vi "CR-导丝颗粒物检测2.vi"(8 "error in (no error)":errorcluster caption="错误输入（无错误）", 11 "名称或相对路径":string="Template Program") -> (0 "error in (no error) 2":errorcluster caption="错误输入（无错误）")   [LabVIEW 2017]
uses:
  Global System.vi
  <vilib>/Utility/xml.llb/Write to XML File(string).vi
  Picture/SaveButtom.ctl
  <vilib>/userdefined/High Color/IMAQdx.ctl
panel:
  in  "相机选择":T1="cam0" caption="Session Out CCD3"
  in  "获取图像":bool
  in  "ROI获取":bool
  in  "创建模板":bool
  in  "保存图像":bool
  out "添加的路径":path
  in  "刷新":bool
  in  "测试按钮":bool
  in  "保存按钮":bool
  in  "Main":enum32{"主参数", "模板匹配参数 ", "测试效果"}(tab)
  in  "颗粒物检测2基础参数":T2={"IsNorImage"=TRUE, "Exposure Values"=100289, "ImagePath"=path "C:/Users/hedongpo/Desktop/514-hdp/Alignment Assemble System/Test Picture/B/3.bmp"} caption="参数界面" {"Exposure Values" scale=0.0..200000.0}
  in  "颗粒物检测2参数":T4={"Rectangle"={"Left"=0, "Top"=0, "Right"=0, "Bottom"=0, "Rotation"=0.0}, "Threshold Limits (Threshold 1)"={"Lower value"=6.0, "Upper value"=245.0}, "Keep/Remove Particles "=FALSE, "Connectivity 4/8 (8) "=TRUE, "Selection Values (Particle Filter 1)"=[{"Measurement Parameter"=35, "Range Lower Value"=80.0, "Range Upper Value"=16332.0, "Range"=FALSE, "Measurement Type"=FALSE}], "Corner Options (Feature Detection 1)"={"Detector type"=enum."Harris Corner", "Kernel size"=7, "Min Corner Point Strength"=32.0}, "Pyramid level (Feature Detection 1)"=3, "Method "=2, "Look For"=0, "Method 2"=2, "ROI Descriptor (Clamp (Rake) 1)"={"Global Rectangle"=[162, 394, 420, 1807], "Contours"=[{"ID"=enum."External", "Type"=12, "Coordinates"=[162, 394, 420, 1807, 0]}]}} {"Method" items=["clustering", "entropy", "metric", "moments", "inter-class variance"]; "Look For" items=["Bright Objects", "Dark Objects"]; "Method 2" items=["clustering", "entropy", "metric", "moments", "inter-class variance"]; "ROI Descriptor (Clamp (Rake) 1)"."Contours"."Type" items=["No Selection", "Point", "Line", "Rectangle", "Oval", "Polygon", "Freehand Region", "Annulus", "Unused2", "Unused3", "Broken Line", "Freehand Line", "Rotated Rectangle"]; "Selection Values (Particle Filter 1)"."Measurement Parameter" items=["Center of Mass X", "Center of Mass Y", "First Pixel X", "First Pixel Y", "Bounding Rect Left", "Bounding Rect Top", "Bounding Rect Right", "Bounding Rect Bottom", "Max Feret Diameter Start X", "Max Feret Diameter Start Y", "Max Feret Diameter End X", "Max Feret Diameter End Y", "Max Horiz. Segment Length Left", "Max Horiz. Segment Length Right", "Max Horiz. Segment Length Row", "-", "Bounding Rect Width", "Bounding Rect Height", "Bounding Rect Diagonal", "Perimeter", "Convex Hull Perimeter", "Holes' Perimeter", "Max Feret Diameter", "Equivalent Ellipse Major Axis", "Equivalent Ellipse Minor Axis", "Equivalent Ellipse Minor Axis (Feret)", "Equivalent Rect Long Side", "Equivalent Rect Short Side", "Equivalent Rect Diagonal", "Equivalent Rect Short Side (Feret)", "Average Horiz. Segment Length", "Average Vert. Segment Length", "Hydraulic Radius", "Waddel Disk Diameter", "-", "Area", "Holes' Area", "Particle & Holes' Area", "Convex Hull Area", "Image Area", "-", "Number of Holes", "Number of Horiz. Segments", "Number of Vert. Segments", "-", "Orientation", "Max Feret Diameter Orientation", "-", "% Area/Image Area", "% Area/(Particle & Holes' Area)", "Ratio of Equivalent Ellipse Axes", "Ratio of Equivalent Rect Sides", "-", "Elongation Factor", "Compactness Factor", "Heywood Circularity Factor", "Type Factor", "-", "Sum X", "Sum Y", "Sum XX", "Sum XY", "Sum YY", "Sum XXX", "Sum XXY", "Sum XYY", "Sum YYY", "-", "Moment of Inertia XX", "Moment of Inertia XY", "Moment of Inertia YY", "Moment of Inertia XXX", "Moment of Inertia XXY", "Moment of Inertia XYY", "Moment of Inertia YYY", "Norm. Moment of Inertia XX", "Norm. Moment of Inertia XY", "Norm. Moment of Inertia YY", "Norm. Moment of Inertia XXX", "Norm. Moment of Inertia XXY", "Norm. Moment of Inertia XYY", "Norm. Moment of Inertia YYY", "Hu Moment 1", "Hu Moment 2", "Hu Moment 3", "Hu Moment 4", "Hu Moment 5", "Hu Moment 6", "Hu Moment 7"]; "Rectangle"."Rotation" min=-90.0 max=90.0 step=1.0 format="%.2f"; "Rectangle"."Left" scale=0.0..1024.0; "Rectangle"."Right" scale=0.0..1024.0}
  in  "Feature Points Strength":string[][](table)
  out "原始图像":T5(plugin-control)
  out "颗粒物有无显示":bool
  out "Number of Features Found":i32
  in  "颗粒物个数阈值":i32
  out "路径输出":path
  in  "Vision Paramter Save Buttom":T6
  out "system time":string
  in  "取消按钮":bool
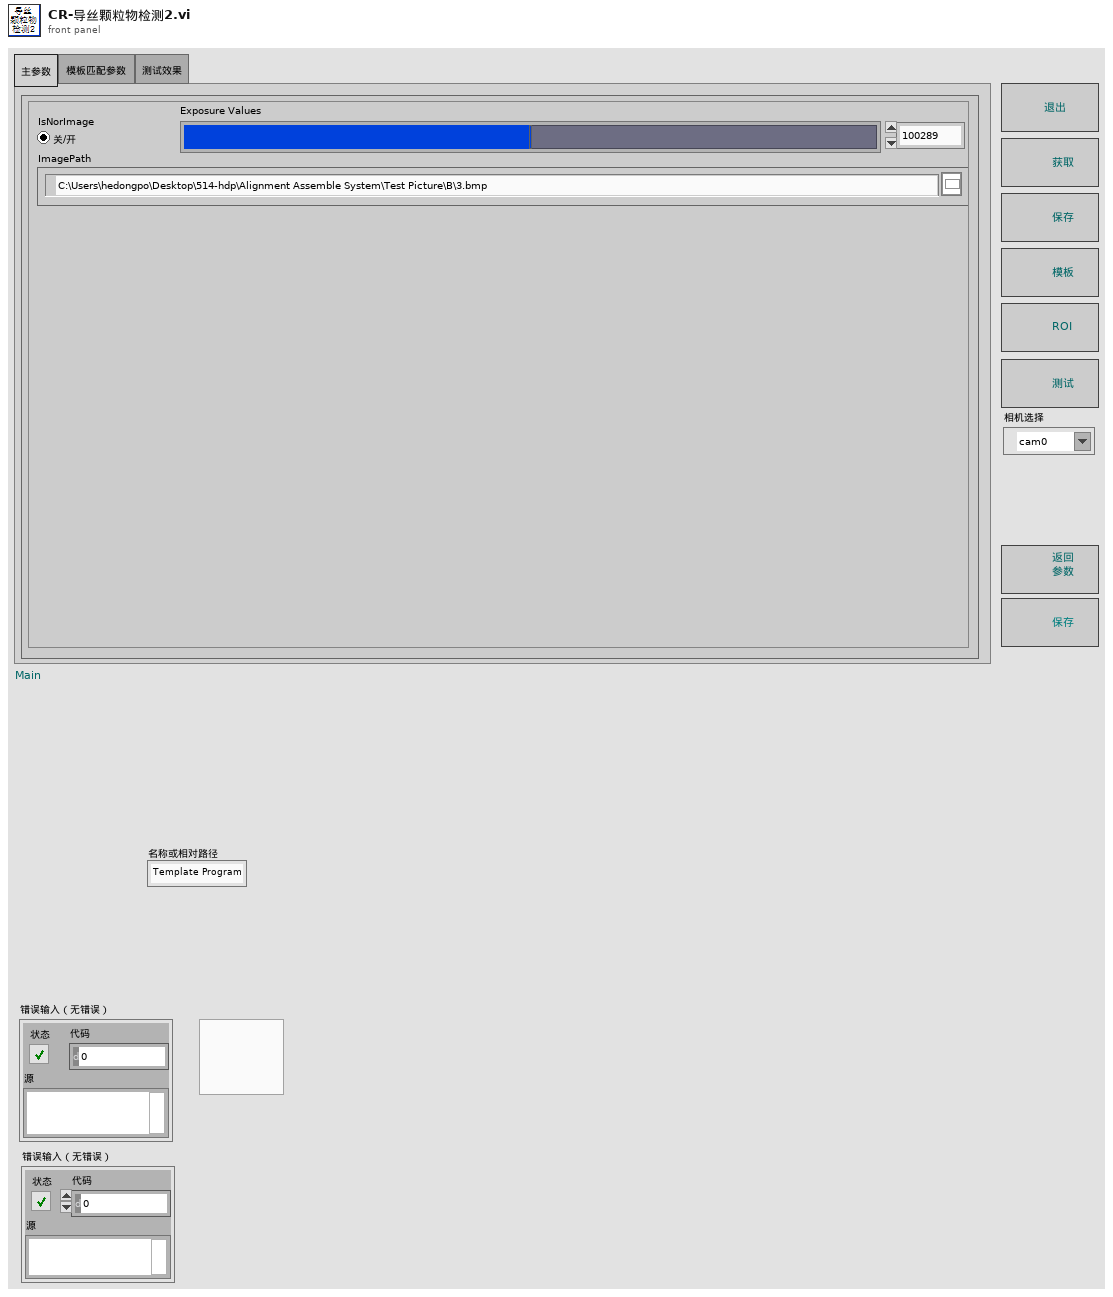
[diagram p1: front panel]
types:
  T1 = typedef "IMAQdx.ctl" = refnum<k21>
  T2 = cluster{"IsNorImage":bool, "Exposure Values":u32, "ImagePath":path}
  T3 = typedef "IMAQ Rectangle" = cluster{"Left":i32, "Top":i32, "Right":i32, "Bottom":i32, "Rotation":dbl}
  T4 = cluster{"Rectangle":T3, "Threshold Limits (Threshold 1)":cluster{"Lower value":sgl, "Upper value":sgl}, "Keep/Remove Particles ":bool, "Connectivity 4/8 (8) ":bool, "Selection Values (Particle Filter 1)":cluster{"Measurement Parameter":i32, "Range Lower Value":dbl, "Range Upper Value":dbl, "Range":bool, "Measurement Type":bool}[], "Corner Options (Feature Detection 1)":cluster{"Detector type":enum32{"Harris Corner", "Shi-Tomasi Corner"}, "Kernel size":i32, "Min Corner Point Strength":dbl}, "Pyramid level (Feature Detection 1)":u32, "Method ":i32, "Look For":u32, "Method 2":i32, "ROI Descriptor (Clamp (Rake) 1)":cluster{"Global Rectangle":i32[], "Contours":cluster{"ID":enum32{"External", "Internal"}, "Type":u32, "Coordinates":i32[]}[]}}
  T5 = typedef "IMAQ Image.ctl" = refnum<image>
  T6 = typedef "SaveButtom.ctl" = bool
  T7 = cluster{"index":i32, "this vi":refnum<vi>, "error out":errorcluster}
  T8 = cluster{"master data":string, "priority":u16, "secondary data":string[]}
  T9 = cluster{"case name":string[], "queue array":refnum<queue>[]}
  T10 = cluster{"Global Rectangle":i32[], "Contours":cluster{"Contour Type":u32, "ROI Type":u32, "Points":i32[]}[]}
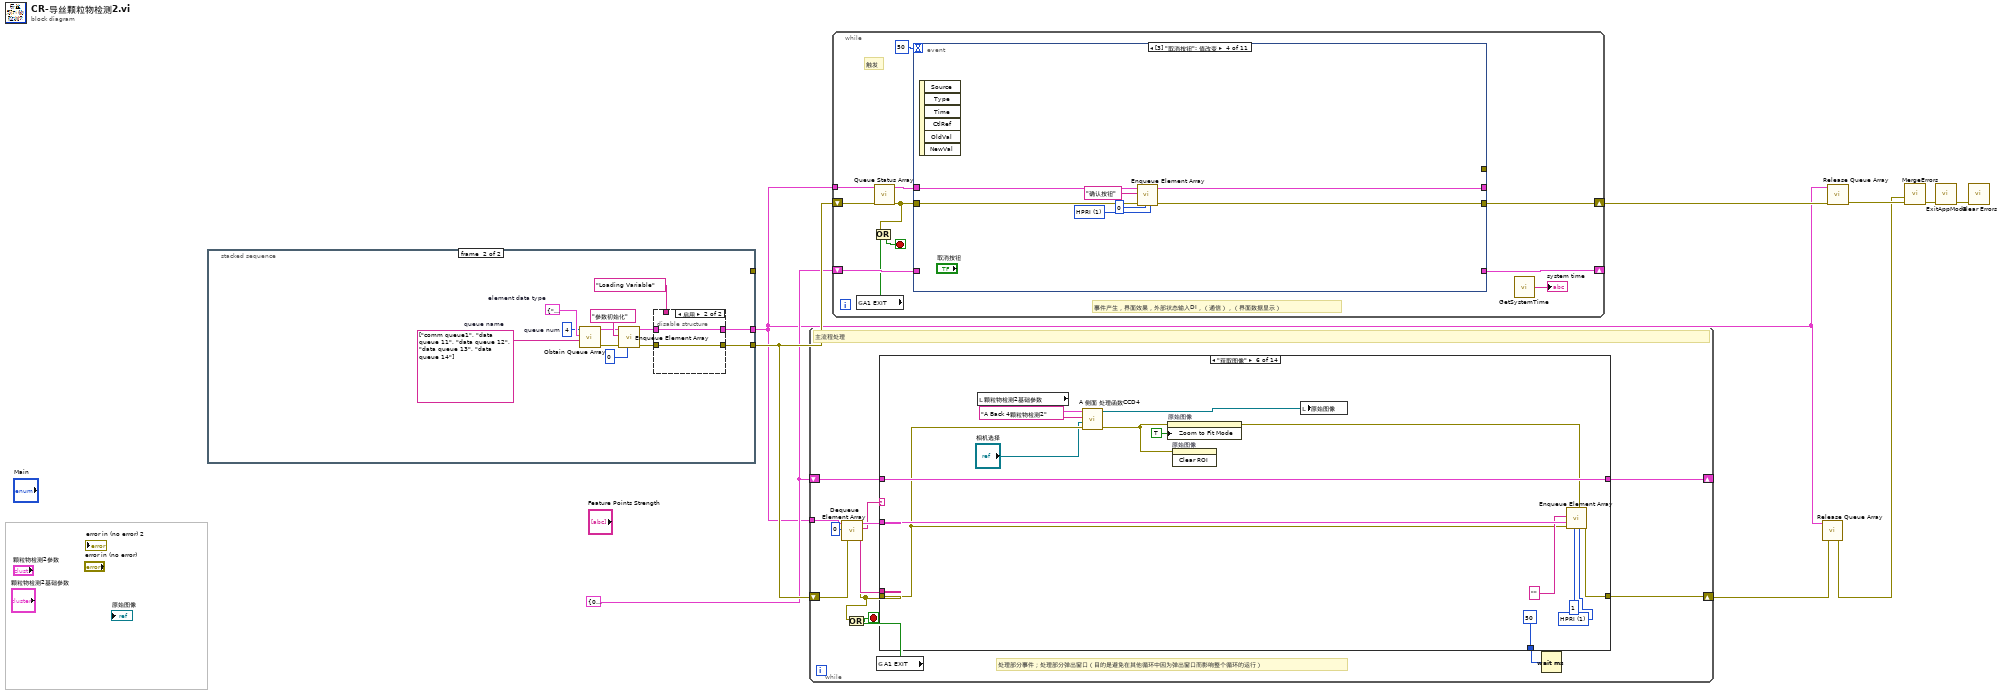
[diagram p0: block diagram]
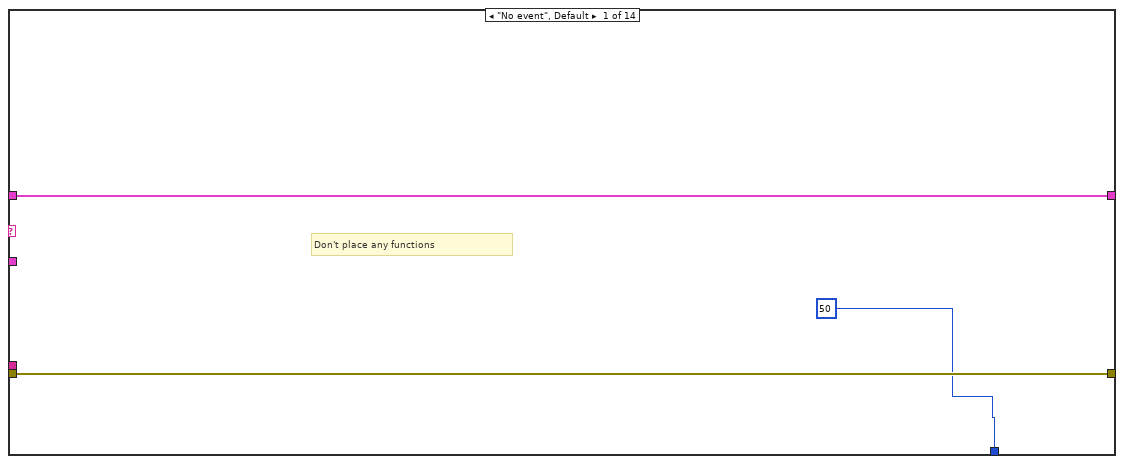
[diagram p2: hidden frame]
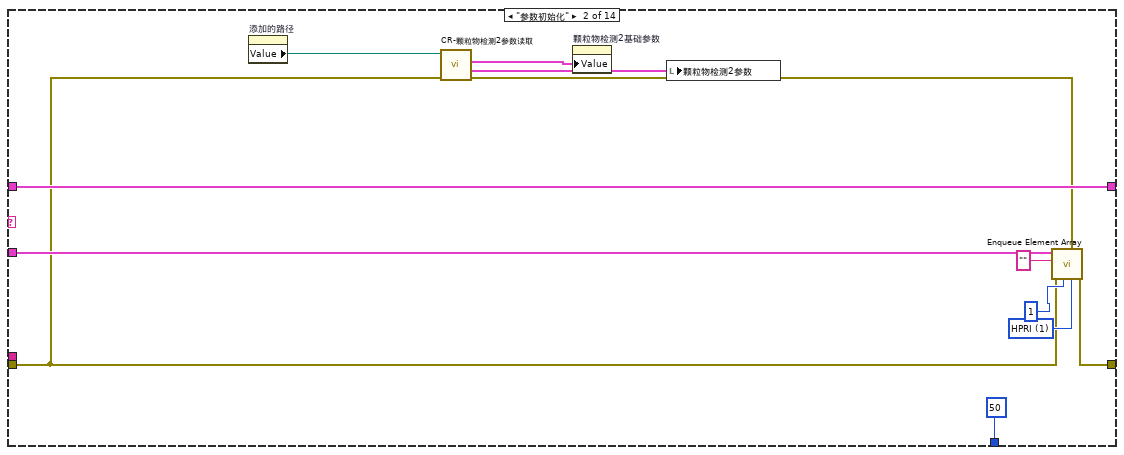
[diagram p3: hidden frame]
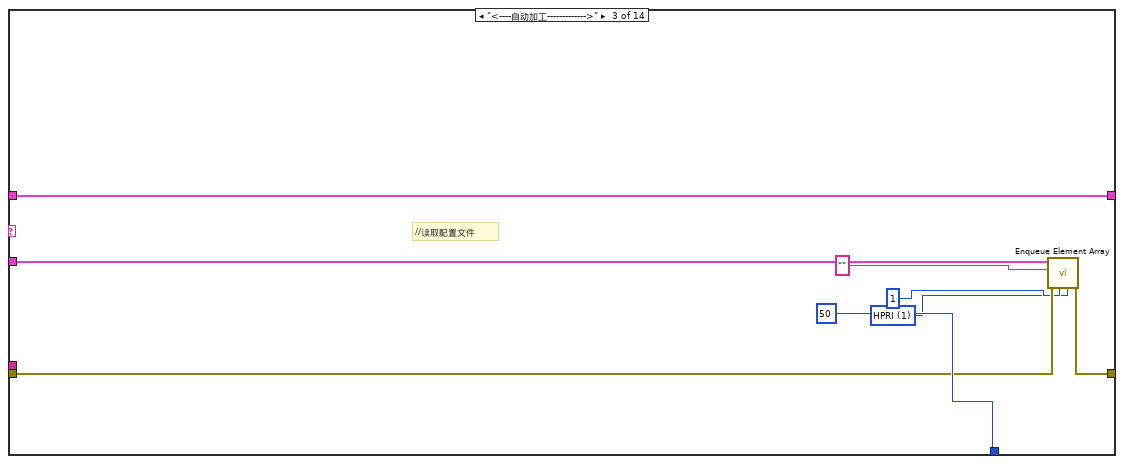
[diagram p4: hidden frame]
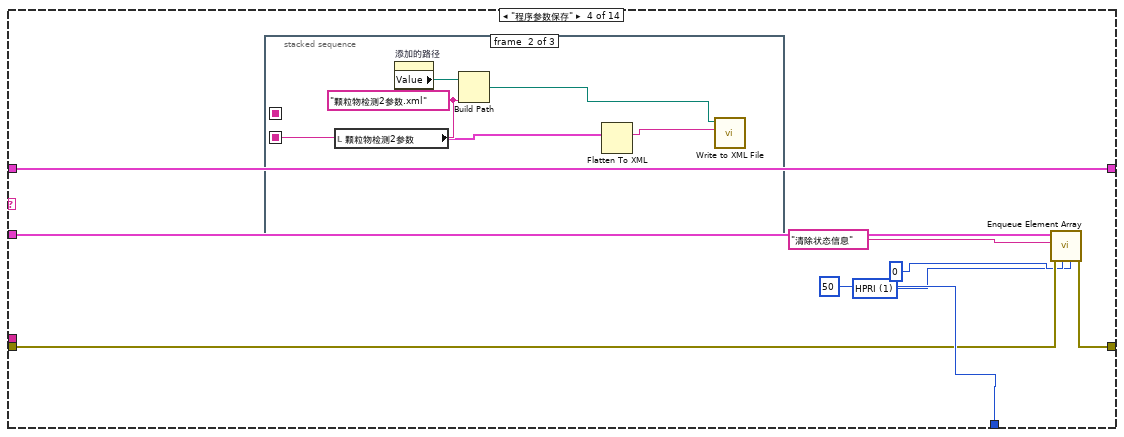
[diagram p5: hidden frame]
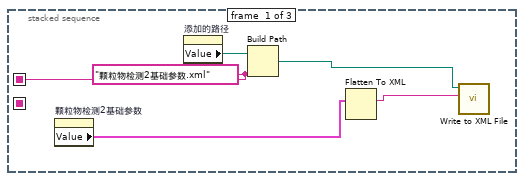
[diagram p6: hidden frame]
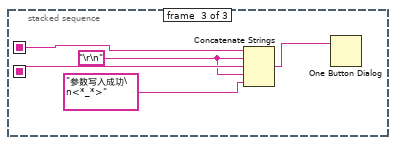
[diagram p7: hidden frame]
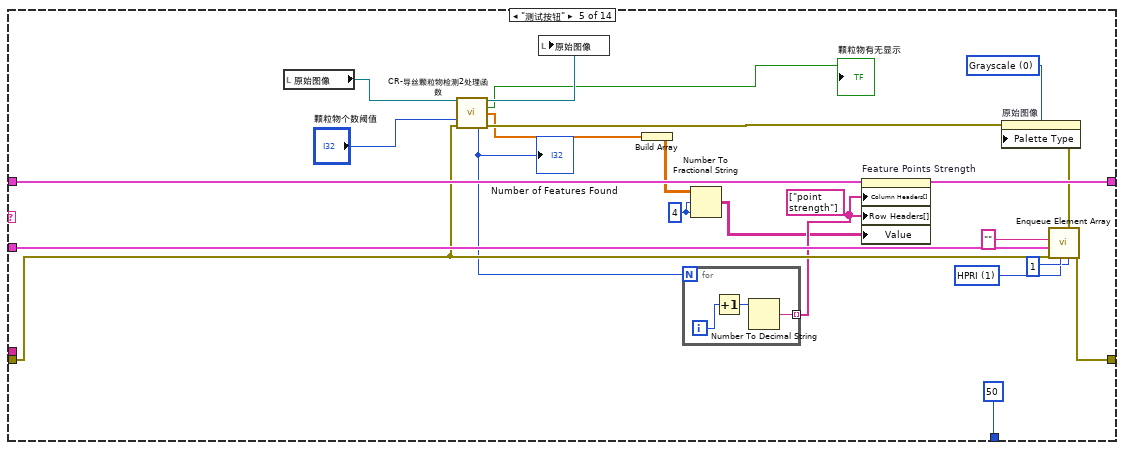
[diagram p8: hidden frame]
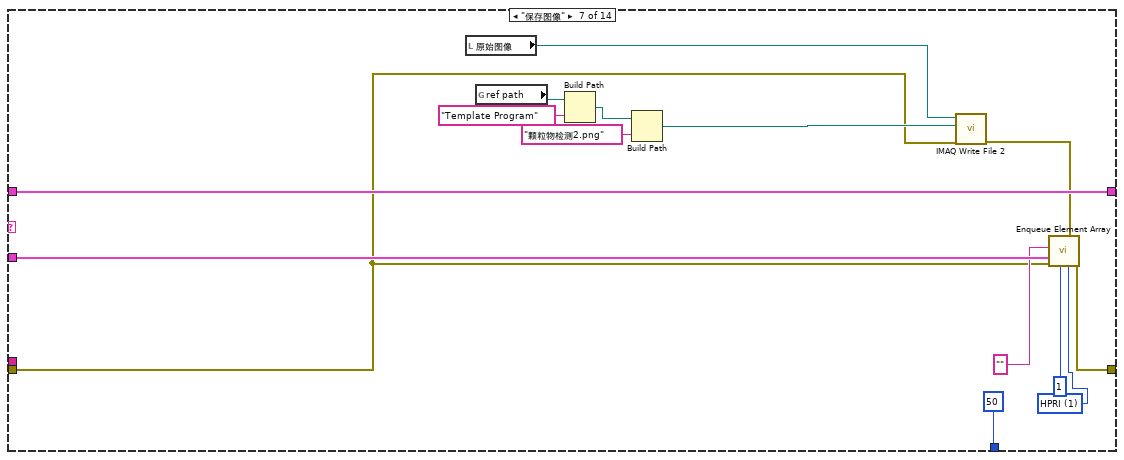
[diagram p9: hidden frame]
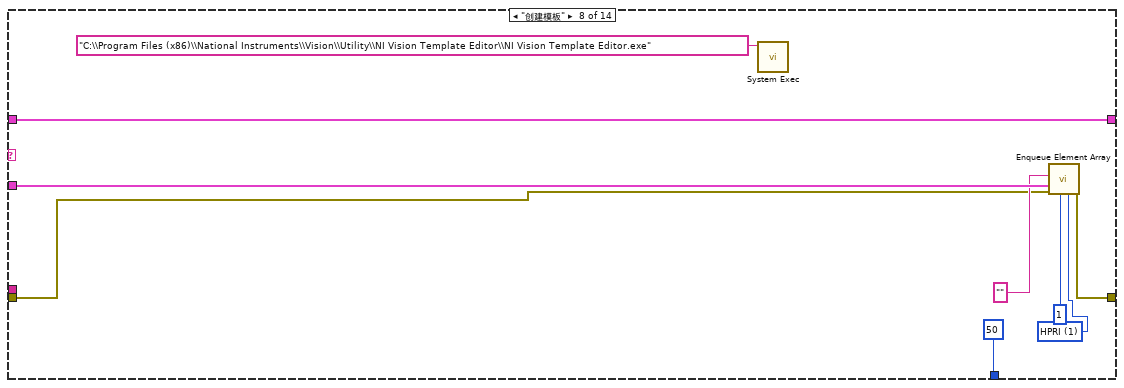
[diagram p10: hidden frame]
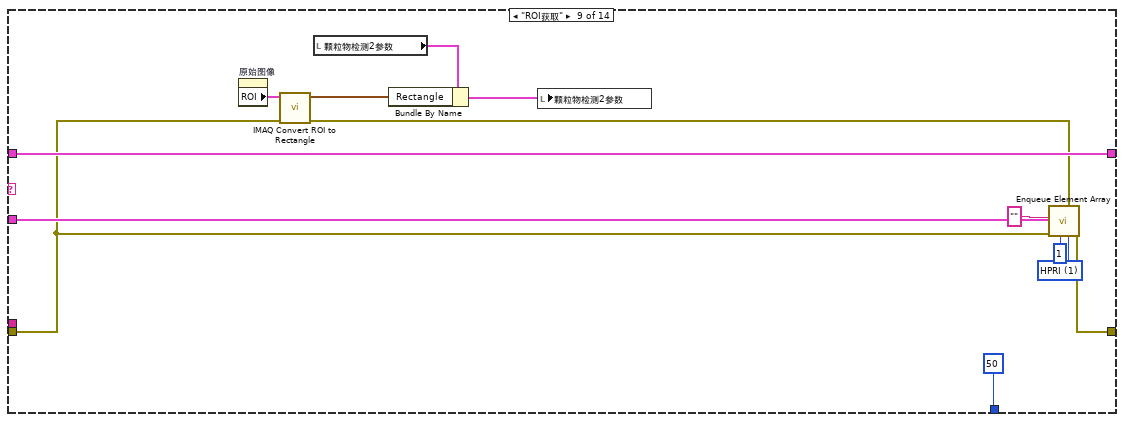
[diagram p11: hidden frame]
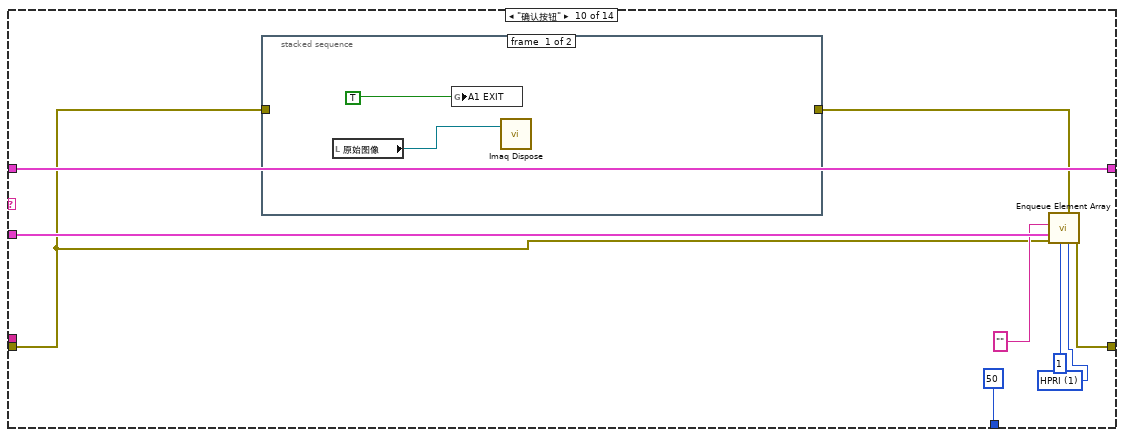
[diagram p12: hidden frame]
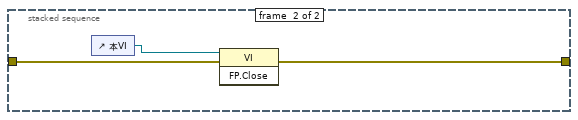
[diagram p13: hidden frame]
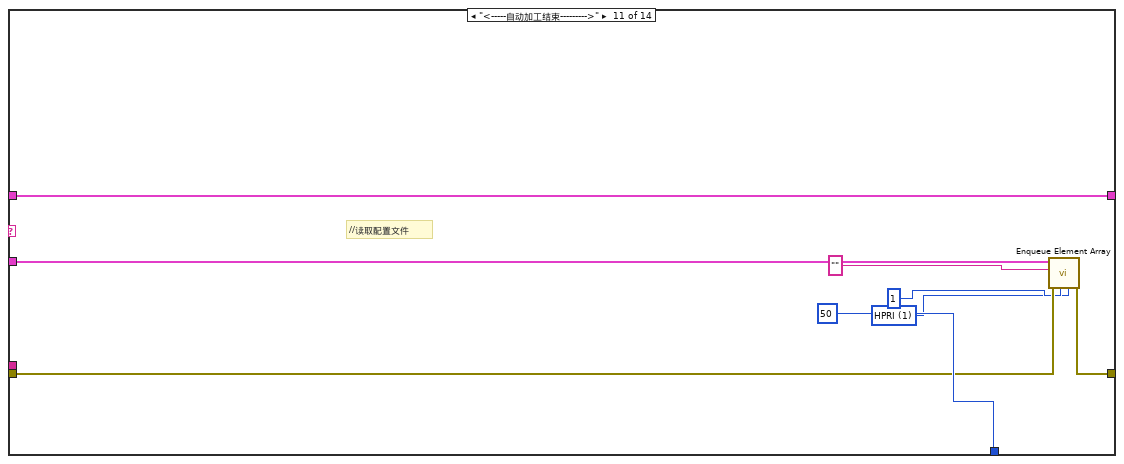
[diagram p14: hidden frame]
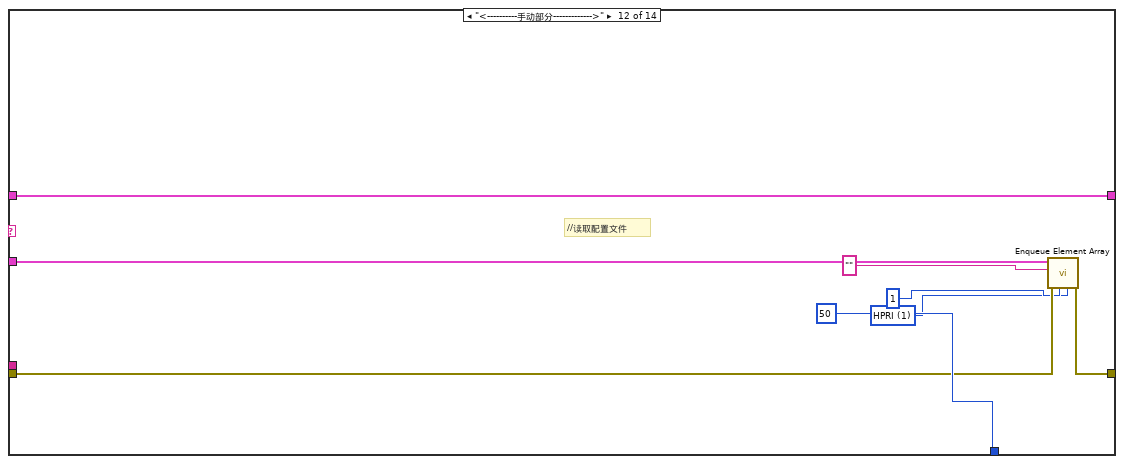
[diagram p15: hidden frame]
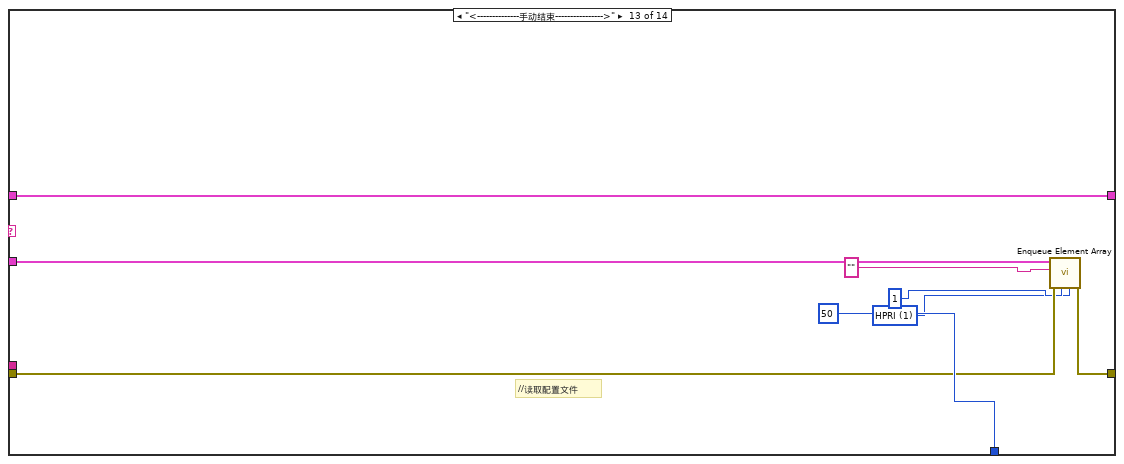
[diagram p16: hidden frame]
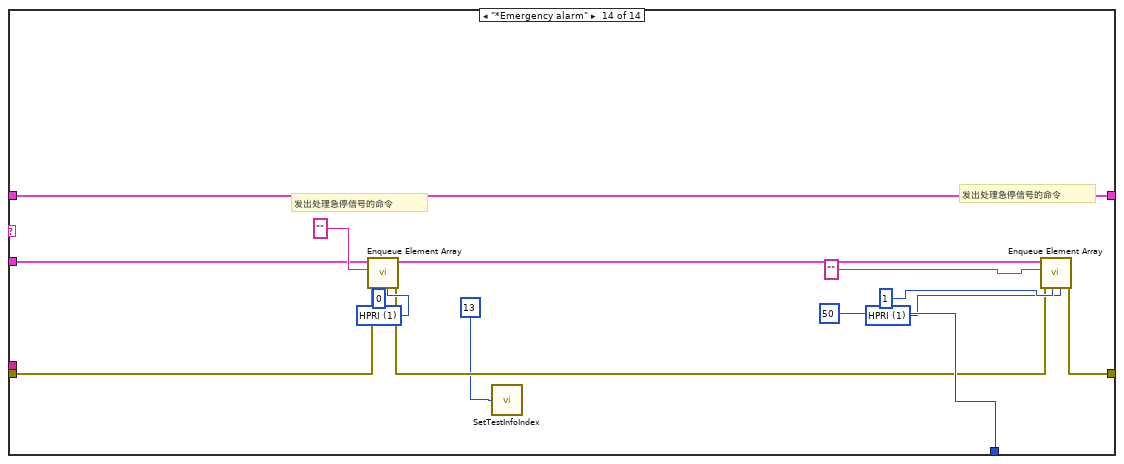
[diagram p17: hidden frame]
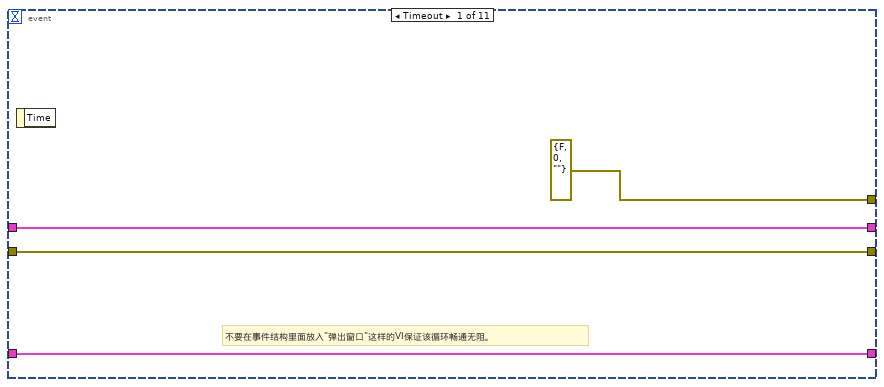
[diagram p18: hidden frame]
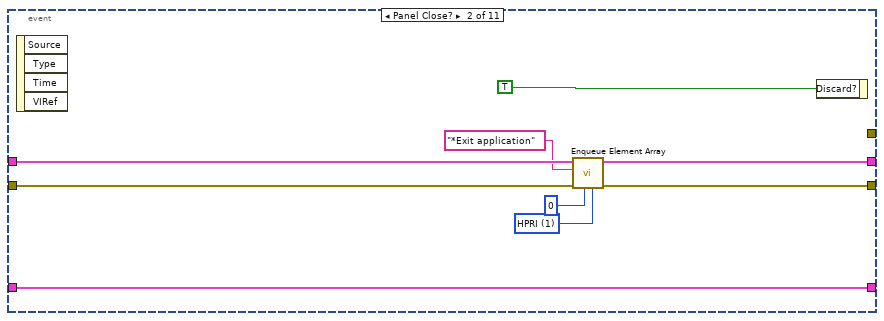
[diagram p19: hidden frame]
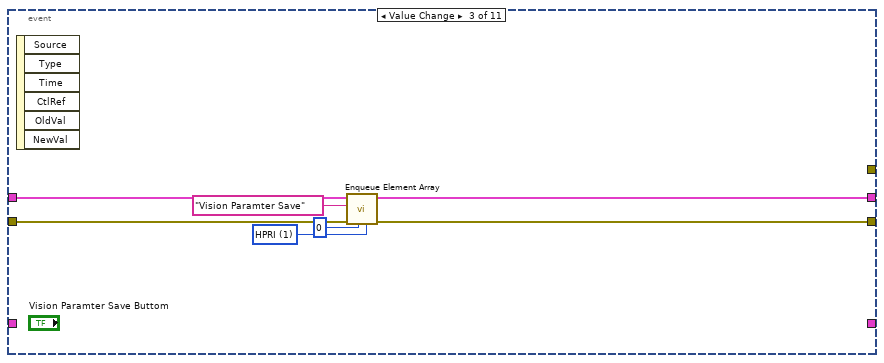
[diagram p20: hidden frame]
diagram:
  w4 = T7 {"index"=0, "this vi"=refnum, "error out"={"status"=FALSE, "code"=0, "source"=""}} ("parameter buffer")
  n1 = stacked-sequence {
    tunnel: [w15 _] -> _
    tunnel: [_ w19] -> w5
    tunnel: [_ w18] -> w1
    frame #0 {
      n2 = global read "Global System.vi" "ref path"() -> (w13:path)
      n3 = Build Path(base path=w13, name or relative path="Template Program" ("名称或相对路径")) -> (appended path=w11:path)
      n4 = property on="Main" class="TabCtl (严格)"("Value"=enum32{"主参数", "模板匹配参数 ", "测试效果"}."主参数" ("Main")) -> ()  [unwired: 2 in, 2 out]
      n5 = Build Path(base path=w11, name or relative path="名称或相对路径") -> (appended path=w17:path)
      "添加的路径" <- w17
      n6 = List Folder(path=w17) -> (path out=→"路径输出":path, error out=w15:errorcluster)  [unwired: 3 in, 2 out]
    }
    frame #1 {
      w27 = string[] ["comm queue1", "data queue 11", "data queue 12", "data queue 13", "data queue 14"]  # queue name
      w28 = 4  # queue num
      w29 = T8 {"master data"="", "priority"=0, "secondary data"=[]}  # element data type
      n7 = call "Obtain Queue Array.vi"("queue name"=w27, "element data type"=w29, "queue num"=w28) -> ("error out"=w23:errorcluster, "queue out"=w24:T9)  [unwired: 2 in, 1 out]
      n8 = call "Enqueue Element Array.vi"("queue index"=0, "error in"=w23, "master data"="参数初始化", "queue in"=w24) -> ("error out"=w22:errorcluster, "queue out"=w21:T9)  [unwired: 6 in]
      n9 = disable-structure shown="启用" {
        disable-tunnel: w22 -> [w35 w36]
        disable-tunnel: w21 -> [w34 w37]
        disable-tunnel: "Loading Variable" ("master data") -> [w33 _]
        disable-tunnel: [w31 w36] -> w19
        disable-tunnel: [w30 w37] -> w18
        frame Disabled {
          n10 = call "Enqueue Element Array.vi"("queue index"=12, "error in"=w35, "master data"=w33, "queue in"=w34) -> ("error out"=w31:errorcluster, "queue out"=w30:T9)  [unwired: 6 in]
        }
        frame Enabled {
        }
      }
    }
  }
  n11 = while {
    shift-right: [w50] -> w3
    shift-left: w5 -> [w41]
    shift-right: [w47] -> _
    shift-left: w4 -> [w48]
    tunnel: w1 -> [w43]
    stop <- w38 stop-if-true
    # "处理部分事件；处理部分弹出窗口（目的是避免在其他循环中因为弹出窗口而影响整个循环的运行）"
    # "主流程处理"
    n12 = call "Dequeue Element Array.vi"("queue in"=w43, "queue index"=0, "error in"=w41) -> ("queue out"=w46:T9, "master data"=w45:string, "secondary data"=w44:string[], "error out"=w40:errorcluster)  [unwired: 2 in, 1 out]
    n13 = global read "Global System.vi" "A1 EXIT"() -> (w39:bool)
    n14 = Or(x=w40, y=w39) -> (x .or. y?=w38:bool)
    n15 = case shown="\"获取图像\"" w45 {
      tunnel: w46 -> [_ w64 w72 w74 w116 w134 w149 w158 w171 w180 w193 w201 w209 w215]
      tunnel: w40 -> [w52 w57 w68 w78 w110 w125 w136 w152 w164 w174 w189 w197 w205 w212]
      tunnel: [w52 w63 w71 w80 w115 w133 w148 w157 w170 w179 w192 w200 w208 w223] -> w50
      tunnel: [50 50 50 50 50 50 50 50 50 50 50 50 50 50] -> w49
      tunnel: w48 -> [w53 w59 w69 w75 w111 w129 w144 w153 w166 w175 w190 w198 w206 w221]
      tunnel: [w53 w59 w69 w75 w111 w129 w144 w153 w166 w175 w190 w198 w206 w221] -> w47
      tunnel: w44 -> [_ _ _ _ _ _ _ _ _ _ _ _ _ _]
      frame "No event", Default {
        # "Don't place any functions"
      }
      frame "参数初始化" {
        w60 = u16 1 items=["HPRI"=1, "LPRI"=0] ("priority")
        n16 = property on="添加的路径" class="Path"() -> ("Value"=w58:path)  [unwired: 2 in, 2 out]
        n17 = call "CR-颗粒物检测2参数读取.vi"("error in (no error)"=w57, "基路径"=w58) -> ("error out"=w54:errorcluster, "颗粒物检测2参数"=w56:T4, "颗粒物检测2基础参数"=w55:T2)  [unwired: 6 in]
        n18 = property on="颗粒物检测2基础参数" class="Clust (严格)"("Value"=w55) -> ()  [unwired: 2 in, 2 out]
        n19 = local write "颗粒物检测2参数"(w56) -> ()
        n20 = call "Enqueue Element Array.vi"("priority"=w60, "device error in"=w54, "queue index"=1, "error in"=w57, "master data"="" ("Element 1"), "queue in"=w64) -> ("error out"=w63:errorcluster)  [unwired: 4 in, 1 out]
      }
      frame "<----自动加工------------->" {
        w66 = u16 1 items=["HPRI"=1, "LPRI"=0] ("priority")
        # "//读取配置文件"
        n21 = call "Enqueue Element Array.vi"("priority"=w66, "queue index"=1, "error in"=w68, "master data"="" ("Element 1"), "queue in"=w72) -> ("error out"=w71:errorcluster)  [unwired: 5 in, 1 out]
      }
      frame "程序参数保存" {
        w76 = u16 1 items=["HPRI"=1, "LPRI"=0] ("priority")
        n22 = stacked-sequence {
          seq-local: [w82 _ _] -> [_ _ w95]
          seq-local: [_ w88 _] -> [_ _ w93]
          frame #0 {
            w82 = "颗粒物检测2基础参数.xml" ("名称或相对路径")
            n23 = property on="颗粒物检测2基础参数" class="Clust (严格)"() -> ("Value"=w85:T2)  [unwired: 2 in, 2 out]
            n24 = property on="添加的路径" class="Path"() -> ("Value"=w86:path)  [unwired: 2 in, 2 out]
            n25 = Build Path(base path=w86, name or relative path=w82) -> (appended path=w83:path)
            n26 = Flatten To XML(anything=w85) -> (xml string=w84:string)
            n27 = call-poly <vilib>:"Write to XML File.vi"("XML Input"=w84, "XML File Path"=w83) -> ()  [unwired: 7 in, 3 out]
          }
          frame #1 {
            w88 = "颗粒物检测2参数.xml" ("名称或相对路径")
            n28 = local read "颗粒物检测2参数"() -> (w87:T4)
            n29 = property on="添加的路径" class="Path"() -> ("Value"=w91:path)  [unwired: 2 in, 2 out]
            n30 = Build Path(base path=w91, name or relative path=w88) -> (appended path=w89:path)
            n31 = Flatten To XML(anything=w87) -> (xml string=w90:string)
            n32 = call-poly <vilib>:"Write to XML File.vi"("XML Input"=w90, "XML File Path"=w89) -> ()  [unwired: 7 in, 3 out]
          }
          frame #2 {
            w92 = "\r\n"
            n33 = Concatenate Strings(w95, w92, w93, w92, "参数写入成功\n<*_*>" ("消息")) -> (w94:string)
            n34 = One Button Dialog(message=w94) -> ()  [unwired: 1 in, 1 out]
          }
        }
        n35 = call "Enqueue Element Array.vi"("priority"=w76, "queue index"=0, "error in"=w78, "master data"="清除状态信息" ("Element 1"), "queue in"=w74) -> ("error out"=w80:errorcluster)  [unwired: 5 in, 1 out]
      }
      frame "测试按钮" {
        w104 = i16 4 ("精度(6)")
        (unwired) string[] ["point strength"] ("列首字符串[]")
        w106 = u32 0 items=["Grayscale", "Binary", "Gradient", "Rainbow", "Temperature", "User Defined", "Binary 16 Bit", "Gradient 16 Bit", "Rainbow 16 Bit", "Temperature 16 Bit", "User Defined 16 Bit"] ("Palette:Palette Type")
        w112 = u16 1 items=["HPRI"=1, "LPRI"=0] ("priority")
        n36 = local read "原始图像"() -> (w108:T5)
        n37 = call "CR-导丝颗粒物检测2处理函数.vi"("Image in"=w108, "颗粒物个数阈值"="颗粒物个数阈值", "error in (no error)"=w110) -> ("Image out"=w109:T5, "颗粒物有无显示"=→"颗粒物有无显示":bool, "颗粒物大小显示"=w101:dbl[], "Number of Features Found"=w97:i32, "error out"=w107:errorcluster)  [unwired: 7 in, 1 out]
        "Number of Features Found" <- w97
        n38 = local write "原始图像"(w109) -> ()
        n39 = Build Array(w101) -> (w103:dbl[][])
        n40 = for {
          N: w97 -> [_]
          tunnel: [w118] -> w99 mode=indexing
          i -> [w120]
          n41 = Increment(x=w120) -> (x+1=w119:i32)
          n42 = Number To Decimal String(number=w119) -> (decimal integer string=w118:string)  [unwired: 1 in]
        }
        n43 = Number To Fractional String(number=w103, width (-)=w104, precision (6)=w104) -> (F-format string=w98:string[][])  [unwired: 1 in]
        n44 = property on="Feature Points Strength" class="Tbl (严格)"("Column Headers[]"=w99, "Row Headers[]"=w99, "Value"=w98) -> ()  [unwired: 2 in, 2 out]
        n45 = property on="原始图像" class="ImageControl"(error in=w107, "Palette Type"=w106) -> (error out=w105:errorcluster)  [unwired: 1 in, 1 out]
        n46 = call "Enqueue Element Array.vi"("priority"=w112, "device error in"=w105, "queue index"=1, "error in"=w110, "master data"="" ("Element 1"), "queue in"=w116) -> ("error out"=w115:errorcluster)  [unwired: 4 in, 1 out]
      }
      frame "获取图像" {
        w130 = u16 1 items=["HPRI"=1, "LPRI"=0] ("priority")
        n47 = local read "颗粒物检测2基础参数"() -> (w127:T2)
        n48 = call "A 侧面 处理函数CCD4.vi"("error in (no error)"=w125, "相机选择"="相机选择", "New Image"="A Back 4颗粒物检测2" ("Image Name"), "ParamsUI"=w127) -> ("error out"=w122:errorcluster, "Image out"=w126:T5)  [unwired: 4 in, 2 out]
        n49 = property on="原始图像" class="ImageControl"(error in=w122, "Zoom to Fit Mode"=TRUE) -> (error out=w123:errorcluster)  [unwired: 1 in, 1 out]
        n50 = invoke on="原始图像" class="ImageControl" method="Clear ROI"(error in=w122) -> ()  [unwired: 2 in, 3 out]
        n51 = local write "原始图像"(w126) -> ()
        n52 = call "Enqueue Element Array.vi"("priority"=w130, "device error in"=w123, "queue index"=1, "error in"=w125, "master data"="" ("Element 1"), "queue in"=w134) -> ("error out"=w133:errorcluster)  [unwired: 4 in, 1 out]
      }
      frame "保存图像" {
        w145 = u16 1 items=["HPRI"=1, "LPRI"=0] ("priority")
        n53 = local read "原始图像"() -> (w137:T5)
        n54 = global read "Global System.vi" "ref path"() -> (w143:path)
        n55 = Build Path(base path=w143, name or relative path="Template Program" ("名称或相对路径")) -> (appended path=w141:path)
        n56 = Build Path(base path=w141, name or relative path="颗粒物检测2.png" ("名称或相对路径")) -> (appended path=w139:path)
        n57 = call-poly "IMAQ Write File 2"("error in (no error)"=w136, "File Path"=w139, "Image"=w137) -> ("error out"=w138:errorcluster)  [unwired: 7 in, 1 out]
        n58 = call "Enqueue Element Array.vi"("priority"=w145, "device error in"=w138, "queue index"=1, "error in"=w136, "master data"="" ("Element 1"), "queue in"=w149) -> ("error out"=w148:errorcluster)  [unwired: 4 in, 1 out]
      }
      frame "创建模板" {
        w154 = u16 1 items=["HPRI"=1, "LPRI"=0] ("priority")
        n59 = call <vilib>:"System Exec.vi"("command line"="C:\\Program Files (x86)\\National Instruments\\Vision\\Utility\\NI Vision Template Editor\\NI Vision Template Editor.exe") -> ()  [unwired: 7 in, 4 out]
        n60 = call "Enqueue Element Array.vi"("priority"=w154, "queue index"=1, "error in"=w152, "master data"="" ("Element 1"), "queue in"=w158) -> ("error out"=w157:errorcluster)  [unwired: 5 in, 1 out]
      }
      frame "ROI获取" {
        w167 = u16 1 items=["HPRI"=1, "LPRI"=0] ("priority")
        n61 = property on="原始图像" class="ImageControl"() -> ("ROI"=w165:T10)  [unwired: 2 in, 2 out]
        n62 = call "IMAQ Convert ROI to Rectangle"("error in (no error)"=w164, "ROI Descriptor"=w165) -> ("error out"=w160:errorcluster, "Rectangle"=w162:T3)  [unwired: 7 in]
        n63 = local read "颗粒物检测2参数"() -> (w163:T4)
        n64 = Bundle By Name(cluster=w163, "Rectangle"=w162) -> (w161:T4)
        n65 = local write "颗粒物检测2参数"(w161) -> ()
        n66 = call "Enqueue Element Array.vi"("priority"=w167, "device error in"=w160, "queue index"=1, "error in"=w164, "master data"="" ("Element 1"), "queue in"=w171) -> ("error out"=w170:errorcluster)  [unwired: 4 in, 1 out]
      }
      frame "确认按钮" {
        w176 = u16 1 items=["HPRI"=1, "LPRI"=0] ("priority")
        n67 = stacked-sequence {
          tunnel: w174 -> [_ w185]
          tunnel: [_ w184] -> w173
          frame #0 {
            n68 = local read "原始图像"() -> (w182:T5)
            n69 = global write "Global System.vi" "A1 EXIT"(TRUE ("EXIT")) -> ()
            n70 = call "Imaq Dispose"("Image"=w182) -> ()  [unwired: 5 in, 1 out]
          }
          frame #1 {
            n71 = control-ref of="本VI"() -> (w186:refnum<vi>)
            n72 = invoke class="VI" method="FP.Close"(reference=w186, error in=w185) -> (error out=w184:errorcluster)  [unwired: 1 in, 2 out]
          }
        }
        n73 = call "Enqueue Element Array.vi"("priority"=w176, "device error in"=w173, "queue index"=1, "error in"=w174, "master data"="" ("Element 1"), "queue in"=w180) -> ("error out"=w179:errorcluster)  [unwired: 4 in, 1 out]
      }
      frame "<-----自动加工结束--------->" {
        w187 = u16 1 items=["HPRI"=1, "LPRI"=0] ("priority")
        # "//读取配置文件"
        n74 = call "Enqueue Element Array.vi"("priority"=w187, "queue index"=1, "error in"=w189, "master data"="" ("Element 1"), "queue in"=w193) -> ("error out"=w192:errorcluster)  [unwired: 5 in, 1 out]
      }
      frame "<----------手动部分------------->" {
        w195 = u16 1 items=["HPRI"=1, "LPRI"=0] ("priority")
        # "//读取配置文件"
        n75 = call "Enqueue Element Array.vi"("priority"=w195, "queue index"=1, "error in"=w197, "master data"="" ("Element 1"), "queue in"=w201) -> ("error out"=w200:errorcluster)  [unwired: 5 in, 1 out]
      }
      frame "<--------------手动结束---------------->" {
        w203 = u16 1 items=["HPRI"=1, "LPRI"=0] ("priority")
        # "//读取配置文件"
        n76 = call "Enqueue Element Array.vi"("priority"=w203, "queue index"=1, "error in"=w205, "master data"="" ("Element 1"), "queue in"=w209) -> ("error out"=w208:errorcluster)  [unwired: 5 in, 1 out]
      }
      frame "*Emergency alarm" {
        w218 = u16 1 items=["HPRI"=1, "LPRI"=0] ("priority")
        w219 = u16 1 items=["HPRI"=1, "LPRI"=0] ("priority")
        # "发出处理急停信号的命令"
        # "发出处理急停信号的命令"
        n77 = call "Enqueue Element Array.vi"("priority"=w218, "queue index"=0, "error in"=w212, "master data"="" ("Element 1"), "queue in"=w215) -> ("error out"=w213:errorcluster, "queue out"=w214:T9)  [unwired: 5 in]
        n78 = call "SetTestInfoIndex.vi"("test info index"=13) -> ()
        n79 = call "Enqueue Element Array.vi"("priority"=w219, "queue index"=1, "error in"=w213, "master data"="" ("Element 1"), "queue in"=w214) -> ("error out"=w223:errorcluster)  [unwired: 5 in, 1 out]
      }
    }
    n80 = Wait (ms)(milliseconds to wait=w49) -> ()  [unwired: 1 out]
  }
  n81 = while {
    shift-right: [w228] -> w6
    shift-left: w5 -> [w232]
    shift-right: [w230] -> _
    shift-left: w4 -> [w231]
    tunnel: w1 -> [w234]
    stop <- w225 stop-if-true
    # "触发"
    # "事件产生，界面效果，外部状态输入DI，（通信），（界面数据显示）"
    n82 = global read "Global System.vi" "A1 EXIT"() -> (w226:bool)
    n83 = call "Queue Status Array.vi"("error in (no error)"=w232, "queue in"=w234) -> ("error out"=w227:errorcluster, "queue out"=w229:T9)  [unwired: 4 in]
    n84 = Or(x=w227, y=w226) -> (x .or. y?=w225:bool)
    n85 = event shown="[3] \"取消按钮\": 值改变" {
      selector: _ -> [_ _ _ _ _ _ _ _ _ _ _]
      dyn-events: _ -> [_ _ _ _ _ _ _ _ _ _ _]
      timeout: 50 -> [_ _ _ _ _ _ _ _ _ _ _]
      tunnel: w231 -> [w239 w247 _ _ _ _ _ _ _ _ _]
      tunnel: [w239 w247 _ _ _ _ _ _ _ _ _] -> w230
      tunnel: [errorcluster {"status"=FALSE, "code"=0, "source"=""} ("error out") _ _ _ _ _ _ _ _ _ _] -> _
      tunnel: w229 -> [w237 w246 w252 w259 w266 w274 w281 w288 w296 w304 w312]
      tunnel: w227 -> [w236 w245 w251 w258 w265 w273 w280 w287 w295 w303 w311]
      tunnel: [w236 w244 w249 w256 w263 w271 w278 w285 w293 w301 w309] -> w228
      tunnel: [w237 w243 w250 w257 w264 w272 w279 w286 w294 w302 w310] -> _
      event Timeout {
        # "不要在事件结构里面放入\"弹出窗口\"这样的VI保证该循环畅通无阻。"
        n86 = event-data() -> ()  [unwired: 1 in, 1 out]
      }
      event Panel Close? {
        w241 = u16 1 items=["HPRI"=1, "LPRI"=0] ("priority")
        n87 = event-data() -> ()  [unwired: 1 in, 4 out]
        n88 = call "Enqueue Element Array.vi"("priority"=w241, "queue index"=0, "error in"=w245, "master data"="*Exit application", "queue in"=w246) -> ("error out"=w244:errorcluster, "queue out"=w243:T9)  [unwired: 5 in]
        n89 = event-data("Discard?"=TRUE) -> ()  [unwired: 1 in, 1 out]
      }
      event Value Change {
        w254 = u16 1 items=["HPRI"=1, "LPRI"=0] ("priority")
        n90 = event-data() -> ()  [unwired: 1 in, 6 out]
        n91 = call "Enqueue Element Array.vi"("priority"=w254, "queue index"=0, "error in"=w251, "master data"="Vision Paramter Save", "queue in"=w252) -> ("error out"=w249:errorcluster, "queue out"=w250:T9)  [unwired: 5 in]
      }
      event "取消按钮": Value Change {
        w261 = u16 1 items=["HPRI"=1, "LPRI"=0] ("priority")
        n92 = event-data() -> ()  [unwired: 1 in, 6 out]
        n93 = call "Enqueue Element Array.vi"("priority"=w261, "queue index"=0, "error in"=w258, "master data"="确认按钮", "queue in"=w259) -> ("error out"=w256:errorcluster, "queue out"=w257:T9)  [unwired: 5 in]
      }
      event "保存按钮": Value Change {
        w268 = u16 1 items=["HPRI"=1, "LPRI"=0] ("priority")
        n94 = event-data() -> ()  [unwired: 1 in, 6 out]
        n95 = call "Enqueue Element Array.vi"("priority"=w268, "queue index"=0, "error in"=w265, "master data"="程序参数保存", "queue in"=w266) -> ("error out"=w263:errorcluster, "queue out"=w264:T9)  [unwired: 5 in]
      }
      event "获取图像": Value Change {
        w276 = u16 1 items=["HPRI"=1, "LPRI"=0] ("priority")
        n96 = event-data() -> ()  [unwired: 1 in, 6 out]
        n97 = property on="Main" class="TabCtl (严格)"("Value"=enum32{"主参数", "模板匹配参数 ", "测试效果"}."测试效果" ("Main")) -> ()  [unwired: 2 in, 2 out]
        n98 = call "Enqueue Element Array.vi"("priority"=w276, "queue index"=0, "error in"=w273, "master data"="获取图像", "queue in"=w274) -> ("error out"=w271:errorcluster, "queue out"=w272:T9)  [unwired: 5 in]
      }
      event "保存图像": Value Change {
        w283 = u16 1 items=["HPRI"=1, "LPRI"=0] ("priority")
        n99 = event-data() -> ()  [unwired: 1 in, 6 out]
        n100 = call "Enqueue Element Array.vi"("priority"=w283, "queue index"=0, "error in"=w280, "master data"="保存图像", "queue in"=w281) -> ("error out"=w278:errorcluster, "queue out"=w279:T9)  [unwired: 5 in]
      }
      event "创建模板": Value Change {
        w290 = u16 1 items=["HPRI"=1, "LPRI"=0] ("priority")
        n101 = event-data() -> ()  [unwired: 1 in, 6 out]
        n102 = call "Enqueue Element Array.vi"("priority"=w290, "queue index"=0, "error in"=w287, "master data"="创建模板", "queue in"=w288) -> ("error out"=w285:errorcluster, "queue out"=w286:T9)  [unwired: 5 in]
      }
      event "ROI获取": Value Change {
        w298 = u16 1 items=["HPRI"=1, "LPRI"=0] ("priority")
        n103 = event-data() -> ()  [unwired: 1 in, 6 out]
        n104 = property on="Main" class="TabCtl (严格)"("Value"=enum32{"主参数", "模板匹配参数 ", "测试效果"}."模板匹配参数 " ("Main")) -> ()  [unwired: 2 in, 2 out]
        n105 = call "Enqueue Element Array.vi"("priority"=w298, "queue index"=0, "error in"=w295, "master data"="ROI获取", "queue in"=w296) -> ("error out"=w293:errorcluster, "queue out"=w294:T9)  [unwired: 5 in]
      }
      event "测试按钮": Value Change {
        w306 = u16 1 items=["HPRI"=1, "LPRI"=0] ("priority")
        n106 = event-data() -> ()  [unwired: 1 in, 6 out]
        n107 = property on="Main" class="TabCtl (严格)"("Value"=enum32{"主参数", "模板匹配参数 ", "测试效果"}."测试效果" ("Main")) -> ()  [unwired: 2 in, 2 out]
        n108 = call "Enqueue Element Array.vi"("priority"=w306, "queue index"=0, "error in"=w303, "master data"="测试按钮", "queue in"=w304) -> ("error out"=w301:errorcluster, "queue out"=w302:T9)  [unwired: 5 in]
      }
      event "刷新": Value Change {
        n109 = event-data() -> ()  [unwired: 1 in, 6 out]
        n110 = disable-structure shown="禁用" {
          disable-tunnel: w312 -> [w316 _]
          disable-tunnel: w311 -> [w315 _]
          disable-tunnel: [w314 _] -> w310
          disable-tunnel: [w313 _] -> w309
          frame Disabled {
            w318 = u16 1 items=["HPRI"=1, "LPRI"=0] ("priority")
            # "刷新"
            n111 = call "Enqueue Element Array.vi"("priority"=w318, "queue index"=0, "error in"=w315, "master data"="刷新", "queue in"=w316) -> ("error out"=w313:errorcluster, "queue out"=w314:T9)  [unwired: 5 in]
          }
          frame Enabled {
          }
        }
        n112 = property on="Main" class="TabCtl (严格)"("Value"=enum32{"主参数", "模板匹配参数 ", "测试效果"}."模板匹配参数 " ("Main")) -> ()  [unwired: 2 in, 2 out]
      }
    }
    n113 = call "GetSystemTime.vi"() -> ("date/time string"=→"system time":string)  [unwired: 7 in]
  }
  n114 = call "Release Queue Array.vi"("error in"=w3, "queue in"=w1) -> ("error out"=w2:errorcluster)  [unwired: 2 in, 3 out]
  n115 = call "Release Queue Array.vi"("error in"=w6, "queue in"=w1) -> ("error out"=w9:errorcluster)  [unwired: 2 in, 3 out]
  n116 = call "MergeErrors.vi"("error in 3 (no error)"=w2, "error in 4 (no error)"=w9) -> ("error out"=w8:errorcluster)  [unwired: 6 in]
  n117 = call "ExitAppMode.vi"("error in (no error)"=w8) -> ("error out"=w7:errorcluster)  [unwired: 10 in]
  n118 = call <vilib>:"Clear Errors.vi"("error in (no error)"=w7) -> ()  [unwired: 5 in, 2 out]
